vi "sub_wf-sum.vi"(11 "History Data":waveform(dbl)[][](array[waveform])) -> (0 "error out":errorcluster caption="에러 출력", 2 "high level x4":T1, 3 "sum of wf":waveform(dbl))   [LabVIEW 2013]
uses:
  <vilib>/measure/mascope.llb/Amplitude and Levels 1 chan.vi
  <vilib>/Waveform/WDTOps.llb/WDT Append Waveforms DBL.vi
  <vilib>/measure/NI_MAPro.lvlib
panel:
  out "크기":i32[](array[numeric])
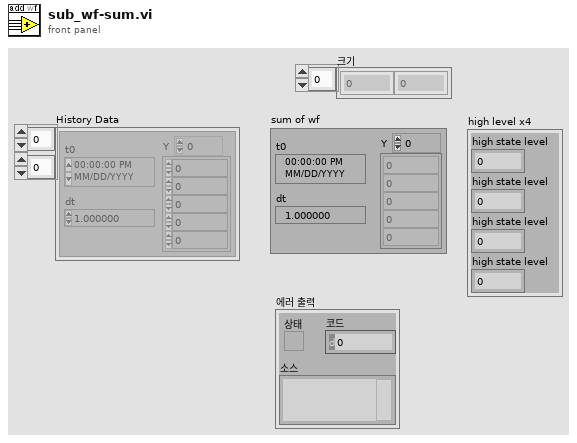
[diagram p1: front panel]
types:
  T1 = cluster{"high state level":dbl, "high state level":dbl, "high state level":dbl, "high state level":dbl}
  T2 = typedef "config_ctl.ctl" = cluster{"Lower Cut-Off":dbl, "Vacuum Trigger level":dbl, "state settings":cluster{"method":enum32{"histogram", "peak", "auto select"}, "histogram size":i32, "histogram method":enum16{"mode"}, "reserved":dbl}, "SPA-300 Setting":cluster{"Bonding force (g)":dbl, "Bonding time (ms)":dbl, "Pickup force (g)":dbl, "Pickup time (ms)":dbl, "Speed":enum16{"Slow", "Fast"}}}
  T3 = cluster{"method":enum32{"histogram", "peak", "auto select"}, "histogram size":i32, "histogram method":enum16{"mode"}, "reserved":dbl}
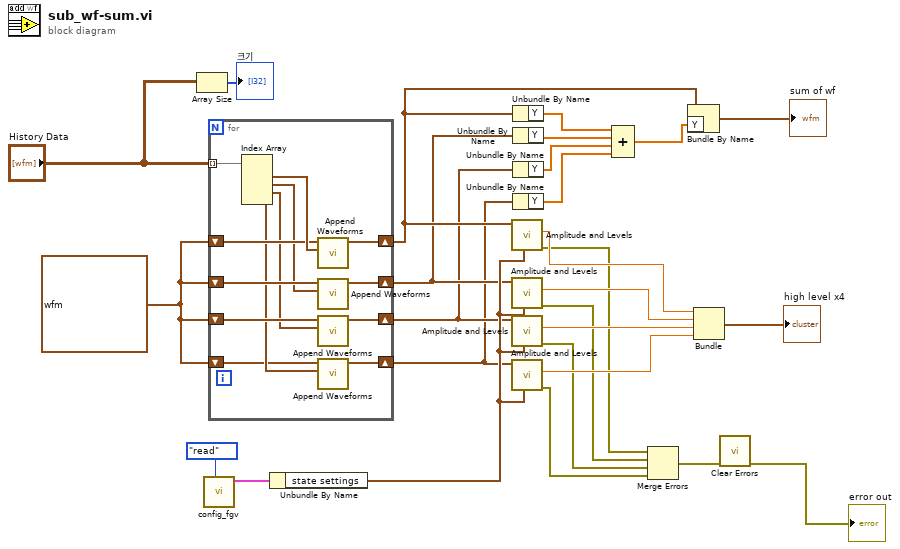
[diagram p0: block diagram]
diagram:
  w18 = waveform(dbl) {"t0"=timestamp(0 s since 1904-01-01), "dt"=0.00062, "Y"=[]} ("원소")
  n1 = Array Size(array="History Data") -> (size(s)=→"크기":i32[])
  n2 = call "config_fgv.vi"("cmd"=enum16{"write", "read", "ini"}."read") -> ("Config out"=w20:T2)  [unwired: 9 in, 1 out]
  n3 = for {
    tunnel: "History Data" -> [w40] mode=indexing
    shift-right: [w39] -> w17
    shift-left: w18 -> [w34]
    shift-right: [w38] -> w16
    shift-left: w18 -> [w33]
    shift-right: [w37] -> w15
    shift-left: w18 -> [w31]
    shift-right: [w36] -> w14
    shift-left: w18 -> [w28]
    n4 = Index Array(array=w40) -> (element #1=w35:waveform(dbl), element #2=w32:waveform(dbl), element #3=w30:waveform(dbl), element #4=w29:waveform(dbl))  [unwired: 4 in]
    n5 = call-poly <vilib>:"Append Waveforms.vi"("waveform B"=w35, "waveform A"=w34) -> ("waveform out"=w39:waveform(dbl))  [unwired: 8 in, 1 out]
    n6 = call-poly <vilib>:"Append Waveforms.vi"("waveform B"=w32, "waveform A"=w33) -> ("waveform out"=w38:waveform(dbl))  [unwired: 8 in, 1 out]
    n7 = call-poly <vilib>:"Append Waveforms.vi"("waveform B"=w30, "waveform A"=w31) -> ("waveform out"=w37:waveform(dbl))  [unwired: 8 in, 1 out]
    n8 = call-poly <vilib>:"Append Waveforms.vi"("waveform B"=w29, "waveform A"=w28) -> ("waveform out"=w36:waveform(dbl))  [unwired: 8 in, 1 out]
  }
  n9 = Unbundle By Name(w20) -> ("state settings"=w22:T3)
  n10 = call-poly <vilib>:"Amplitude and Levels.vi"("state settings"=w22, "signal in"=w17) -> ("error out"=w8:errorcluster, "high state level"=w24:dbl)  [unwired: 6 in, 2 out]
  n11 = call-poly <vilib>:"Amplitude and Levels.vi"("state settings"=w22, "signal in"=w16) -> ("error out"=w7:errorcluster, "high state level"=w25:dbl)  [unwired: 6 in, 2 out]
  n12 = call-poly <vilib>:"Amplitude and Levels.vi"("state settings"=w22, "signal in"=w15) -> ("error out"=w6:errorcluster, "high state level"=w26:dbl)  [unwired: 6 in, 2 out]
  n13 = call-poly <vilib>:"Amplitude and Levels.vi"("state settings"=w22, "signal in"=w14) -> ("error out"=w5:errorcluster, "high state level"=w27:dbl)  [unwired: 6 in, 2 out]
  n14 = Unbundle By Name(w17) -> ("Y"=w12:dbl[])
  n15 = Unbundle By Name(w16) -> ("Y"=w11:dbl[])
  n16 = Unbundle By Name(w15) -> ("Y"=w10:dbl[])
  n17 = Unbundle By Name(w14) -> ("Y"=w9:dbl[])
  n18 = Compound Arithmetic op=ADD(w12, w11, w10, w9) -> (w13:dbl[])
  n19 = Merge Errors(w8, w7, w6, w5) -> (w4:errorcluster)
  n20 = Bundle By Name(cluster=w17, "Y"=w13) -> (→"sum of wf":waveform(dbl))
  n21 = Bundle("high state level"=w24, "high state level"=w25, "high state level"=w26, "high state level"=w27) -> (→"high level x4":T1)  [unwired: 1 in]
  n22 = call <vilib>:"Clear Errors.vi"("error in (no error)"=w4) -> ("error out"=→"error out":errorcluster)  [unwired: 6 in]
